vi "Tell Child Forward.vi"(4 "Alias":string, 6 "Msg":refnum<class "Msg.lvclass">, 7 "Actor in":refnum<class "Actor.lvclass">, 8 "Error in":errorcluster, 9 "Msg Attributes":refnum<data-value>, 10 "Previous Told":bool) -> (0 "Error out":errorcluster, 1 "Told":bool, 2 "Told Or Previous Told":bool, 5 "Actor out":refnum<class "Actor.lvclass">)   [LabVIEW 2020, in "_Template.lvlib" / "Templates.lvlib" / "TEMPLATE jettl Msg.lvlib" / "TEMPLATE.lvlib"]
uses:
  TEMPLATE/TEMPLATE.lvlib
  jettl/jettl/jettl.lvlib
  jettl/jettl/Actor/Actor.lvclass
  jettl/jettl/Relation.ctl
  jettl/jettl/Teller.ctl
  jettl/jettl/Msg Input/Msg Input.lvclass
  jettl/jettl/Msg Output/Msg Output.lvclass
  jettl/jettl/Msg/Msg.lvclass
  jettl/jettl/Msg Attributes.ctl
  jettl/jettl/Transport/Transport.lvclass
  jettl/jettl/Msgs.ctl
  jettl/jettl/Unified Layer.ctl
  jettl/jettl/Actor Attributes.ctl
panel:
  # "This front panel should not be manipulated."
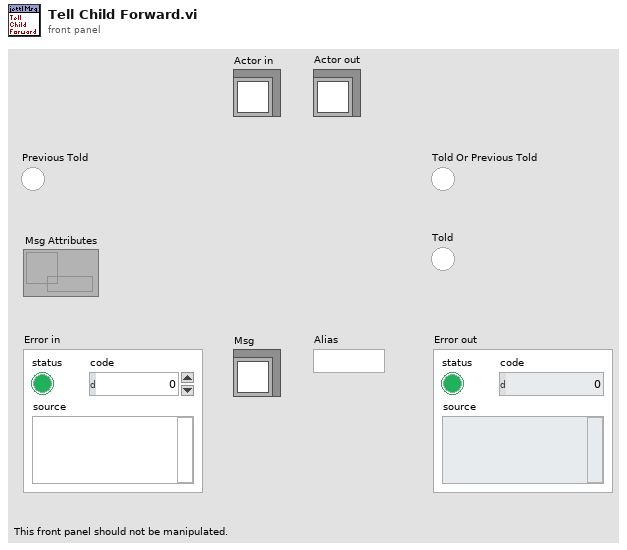
[diagram p1: front panel]
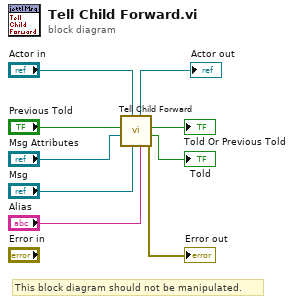
[diagram p0: block diagram]
diagram:
  # "This block diagram should not be manipulated."
  n1 = call "Tell Child Forward.vi"("Alias"="Alias", "Msg"="Msg", "Actor in"="Actor in", "Msg Attributes"="Msg Attributes", "Previous Told"="Previous Told") -> ("Error out"=→"Error out":errorcluster, "Told"=→"Told":bool, "Told Or Previous Told"=→"Told Or Previous Told":bool, "Actor out"=→"Actor out":refnum<class "Actor.lvclass">)  [unwired: 3 in]
